vi "S2C_UpdateDrivers.vi"(8 "Error In":errorcluster, 11 "MenuRef":refnum<k9>) -> (0 "Error Out":errorcluster)   [LabVIEW 2015]
doc: "Toggles the \"Local File\" runtime menu item."
uses:
  Globals/S2C_GlobalMenus.vi
  Core/Command/S2C_CMD_Globals.vi
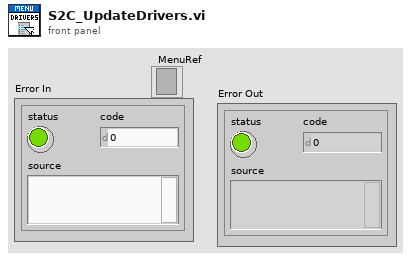
[diagram p1: front panel]
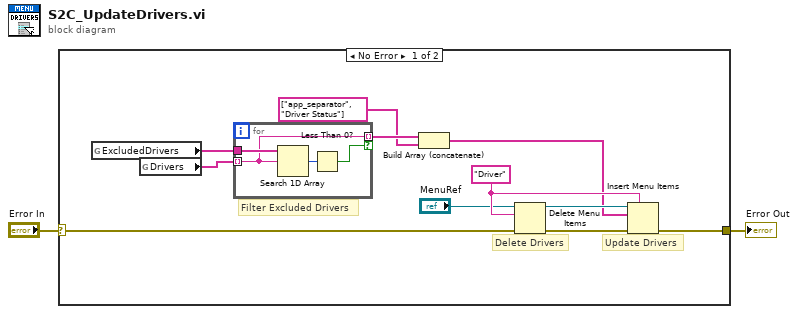
[diagram p0: block diagram]
diagram:
  n1 = case shown="No Error" "Error In" {
    selector: "Error In" -> [w3 w18]
    tunnel: [w10 w18] -> w1
    frame No Error {
      w12 = "Driver" ("item tag")
      # "Update Drivers"
      # "Delete Drivers"
      # "Filter Excluded Drivers"
      n2 = global read "S2C_GlobalMenus.vi" "ExcludedDrivers"() -> (w5:string[])
      n3 = global read "S2C_CMD_Globals.vi" "Drivers"() -> (w4:string[])
      n4 = for {
        tunnel: [w14] -> w8 mode=indexing if=w15
        tunnel: w5 -> [w17]
        tunnel: w4 -> [w14] mode=indexing
        n5 = Search 1D Array(1D array=w17, element=w14) -> (index of element=w16:i32)  [unwired: 1 in]
        n6 = Less Than 0?(x=w16) -> (x < 0?=w15:bool)
      }
      n7 = Build Array (concatenate)(w8, string[] ["app_separator", "Driver Status"]) -> (w6:string[])
      n8 = Delete Menu Items(6:w3, 8:w12, 9:"MenuRef") -> (0:w13:errorcluster, 3:w11:refnum<k9>)  [unwired: 1 in]
      n9 = Insert Menu Items(5:w12, 6:w13, 8:w6, 9:w11) -> (0:w10:errorcluster)  [unwired: 2 in, 2 out]
    }
    frame Error {
    }
  }
  "Error Out" <- w1
